vi "BOOLEAN OPERATIONS.vi"() -> ()   [LabVIEW 2025]
panel:
  out "XNOR":bool
  out "XOR":bool
  out "NOR":bool
  out "NAND2":bool
  out "NOT":bool
  out "OR":bool
  out "AND":bool
  in  "B":bool
  in  "A":bool
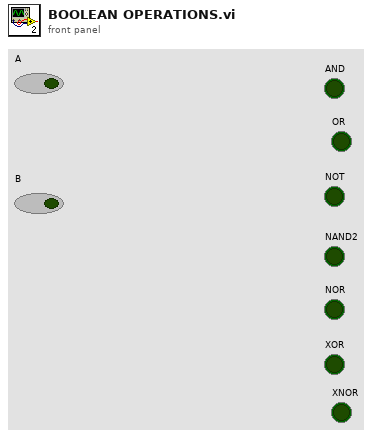
[diagram p1: front panel]
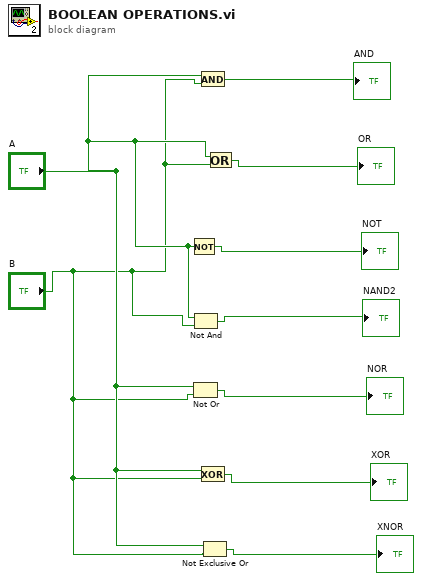
[diagram p0: block diagram]
diagram:
  n1 = Not(x="A") -> (.not. x?=→"NOT":bool)
  n2 = Not Or(1:"B", 2:"A") -> (0:→"NOR":bool)
  n3 = Not And(1:"B", 2:"A") -> (0:→"NAND2":bool)
  n4 = And(x="A", y="B") -> (x .and. y?=→"AND":bool)
  n5 = Exclusive Or(1:"B", 2:"A") -> (0:→"XOR":bool)
  n6 = Not Exclusive Or(1:"B", 2:"A") -> (0:→"XNOR":bool)
  n7 = Or(x="A", y="B") -> (x .or. y?=→"OR":bool)
